vi "LuaVIEW Register and Set Module Function.vi"(0 "module refnum":refnum<vi>, 1 "export table (set as global)":string, 2 "table (set as global)":string, 5 "LuaVIEW reference in":T1, 7 "index":i32, 9 "synopsis":string, 11 "error in (no error)":errorcluster) -> (6 "LuaVIEW reference out":T1, 15 "error out":errorcluster)   [LabVIEW 2012]
doc: "Registers a module function with the LuaVIEW state's private function registry and sets the function as part of the state's variable space so that it can be called by name. When the function is to be exported, as denoted by an exclamation mark prefix to its synopsis, it is also registered with the public function registry. If an exported module function of that name and table is already present, it will be replaced. This implies that the module or module instance called via an exported module function can change while a script is running. Replace exports only when they offer equivalent functionality."
uses:
  typedefs/t_LuaVIEW Reference.ctl
  typedefs/et_LuaVIEW CIN Actions.ctl
  typedefs/t_LuaVIEW CIN Spinlocked Actions.ctl
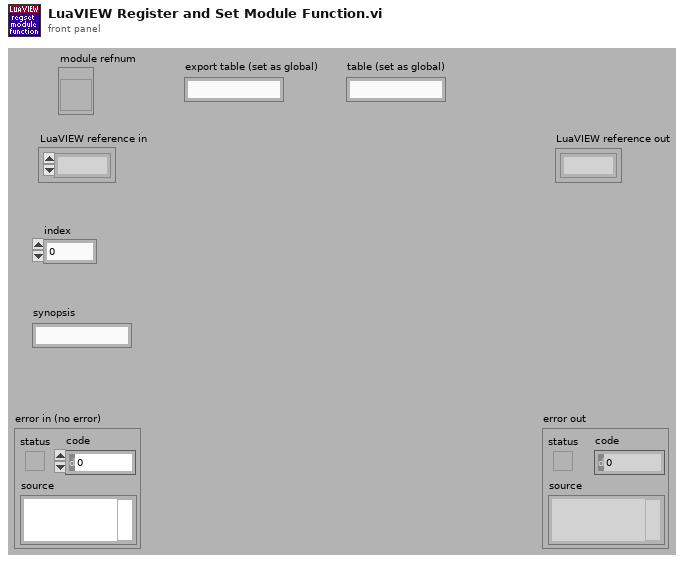
[diagram p1: front panel]
types:
  T1 = typedef "t_LuaVIEW Reference.ctl" = refnum<k1>
  T2 = typedef "et_LuaVIEW CIN Actions.ctl" = enum16{"checksynopsis", "_open", "_registerpublic", "_registerexport", "__never_an_error_result_ns", "luaversion", "cinversion", "_totals", "_taskcount", "pathological", "_unregnextpublic", "registryusecount", "__per_state_actions", "regsetprivate", "regsetindex", "regsetmodule", "_revokeexports", "_usepublic", "prepare", "compile", "execute", "call", "unregstaterefs", "_close", "pullboolean", "pullnumber", "pullI8", "pullU8", "pullI16", "pullU16", "pullI32", "pullU32", "pullobject", "pullrefnum", "pullstring", "pullflat", "pushflat", "pushobject", "getattribute", "setattribute", "stacktostring", "_startyieldtest", "_endyieldtest", "_pollprintbuffer", "__never_an_error_result_ps", "_pollexport", "setclone", "forcecleanup", "gettop", "clearstack", "insert", "pushboolean", "pushnumber", "pushrefnum", "pushstring", "pushnil", "pushvalue", "gettaskref", "settaskref"}
  T3 = typedef "t_LuaVIEW CIN Spinlocked Actions.ctl" = enum16{"totals", "taskcount", "open", "registerpublic", "registerexport", "revokeexports", "unregnextpublic", "usepublic", "pollexport", "close", "startyieldtest", "endyieldtest", "pollprintbuffer"}
  T4 = typedef "et_LuaVIEW CIN Results.ctl" = enum16{"OK", "error", "main", "call", "clonecall", "modulecall", "exportcall", "index", "yield"}
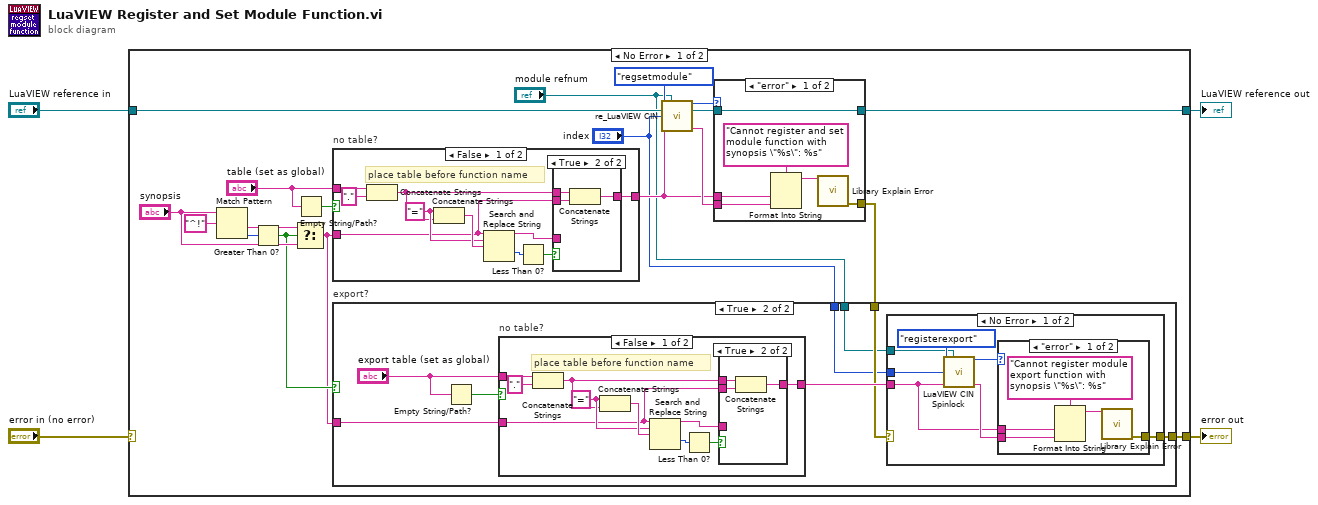
[diagram p0: block diagram]
diagram:
  n1 = case shown="No Error" "error in (no error)" {
    selector: "error in (no error)" -> [_ w83]
    tunnel: [w19 w84] -> w4
    tunnel: "LuaVIEW reference in" -> [w18 w84]
    tunnel: [w7 w83] -> w1
    frame No Error {
      n2 = Match Pattern(string="synopsis", regular expression="^!") -> (after substring=w12:string, offset past match=w13:i32)  [unwired: 1 in, 2 out]
      n3 = Greater Than 0?(x=w13) -> (x > 0?=w10:bool)
      n4 = Select(t=w12, s=w10, f="synopsis") -> (s? t:f=w9:string)
      n5 = Empty String/Path?(string/path="table (set as global)") -> (empty?=w16:bool)
      n6 = case "no table?" shown="False" w16 {
        tunnel: "table (set as global)" -> [w70 _]
        tunnel: w9 -> [w62 w75]
        tunnel: [w63 w75] -> w15
        frame False {
          w67 = "=" ("string")
          # "place table before function name"
          n7 = Concatenate Strings(w70, "." ("string")) -> (w61:string)
          n8 = Concatenate Strings(w67, w61) -> (w68:string)
          n9 = Search and Replace String(input string=w62, search string=w67, replace string=w68) -> (result string=w64:string, offset past replacement=w66:i32)  [unwired: 5 in, 2 out]
          n10 = Less Than 0?(x=w66) -> (x < 0?=w65:bool)
          n11 = case shown="True" w65 {
            tunnel: w64 -> [w71 _]
            tunnel: [w71 w72] -> w63
            tunnel: w62 -> [_ w74]
            tunnel: w61 -> [_ w73]
            frame False {
            }
            frame True {
              n12 = Concatenate Strings(w73, w74) -> (w72:string)
            }
          }
        }
        frame True {
        }
      }
      n13 = call "re_LuaVIEW CIN.vi"("action"=et_LuaVIEW_CIN_Actions."regsetmodule", "refnum in"="module refnum", "LuaVIEW reference in"=w18, "index in"="index", "string in"=w15) -> ("result"=w22:T4, "LuaVIEW reference out"=w20:T1, "string out"=w21:string)  [unwired: 4 in, 4 out]
      n14 = case shown="\"error\"" w22 {
        tunnel: w21 -> [w80 _]
        tunnel: [w81 _] -> w8
        tunnel: w15 -> [w79 _]
        tunnel: w20 -> [w76 w82]
        tunnel: [w76 w82] -> w19
        frame "error" {
          n15 = Format Into String(format string="Cannot register and set module function with  synopsis \"%s\": %s", w79, w80) -> (resulting string=w77:string)  [unwired: 2 in, 1 out]
          n16 = call "Library Explain Error.vi"("explanation prefix (none)"=w77) -> ("explained error"=w81:errorcluster)  [unwired: 14 in]
        }
        frame Default {
        }
      }
      n17 = case "export?" shown="True" w10 {
        tunnel: w9 -> [_ w30]
        tunnel: w8 -> [w24 w28]
        tunnel: [w24 w27] -> w7
        tunnel: "index" -> [_ w26]
        tunnel: "module refnum" -> [_ w25]
        frame False {
        }
        frame True {
          n18 = Empty String/Path?(string/path="export table (set as global)") -> (empty?=w32:bool)
          n19 = case "no table?" shown="False" w32 {
            tunnel: "export table (set as global)" -> [w55 _]
            tunnel: w30 -> [w47 w60]
            tunnel: [w48 w60] -> w29
            frame False {
              w52 = "=" ("string")
              # "place table before function name"
              n20 = Concatenate Strings(w55, "." ("string")) -> (w46:string)
              n21 = Concatenate Strings(w52, w46) -> (w53:string)
              n22 = Search and Replace String(input string=w47, search string=w52, replace string=w53) -> (result string=w49:string, offset past replacement=w51:i32)  [unwired: 5 in, 2 out]
              n23 = Less Than 0?(x=w51) -> (x < 0?=w50:bool)
              n24 = case shown="True" w50 {
                tunnel: w49 -> [w56 _]
                tunnel: [w56 w57] -> w48
                tunnel: w47 -> [_ w59]
                tunnel: w46 -> [_ w58]
                frame False {
                }
                frame True {
                  n25 = Concatenate Strings(w58, w59) -> (w57:string)
                }
              }
            }
            frame True {
            }
          }
          n26 = case shown="No Error" w28 {
            selector: w28 -> [_ w45]
            tunnel: w29 -> [w34 _]
            tunnel: [w37 w45] -> w27
            tunnel: w26 -> [w36 _]
            tunnel: w25 -> [w33 _]
            frame No Error {
              n27 = call "LuaVIEW CIN Spinlock.vi"("action"=t_LuaVIEW_CIN_Spinlocked_Actions."registerexport", "refnum in"=w33, "index in"=w36, "string in"=w34) -> ("result"=w38:T4, "string out"=w35:string)  [unwired: 5 in, 5 out]
              n28 = case shown="\"error\"" w38 {
                tunnel: w35 -> [w43 _]
                tunnel: [w44 _] -> w37
                tunnel: w34 -> [w42 _]
                frame "error" {
                  n29 = Format Into String(format string="Cannot register module export function with  synopsis \"%s\": %s", w42, w43) -> (resulting string=w40:string)  [unwired: 2 in, 1 out]
                  n30 = call "Library Explain Error.vi"("explanation prefix (none)"=w40) -> ("explained error"=w44:errorcluster)  [unwired: 14 in]
                }
                frame Default {
                }
              }
            }
            frame Error {
            }
          }
        }
      }
    }
    frame Error {
    }
  }
  "LuaVIEW reference out" <- w4
  "error out" <- w1
